vi "Acquire.vi"(8 "error in (no error)":errorcluster, 11 "ATS9350 in":refnum<class "ATS9350.lvclass">) -> (0 "error out":errorcluster, 3 "ATS9350 out":refnum<class "ATS9350.lvclass">)   [LabVIEW 2014, in "ATS9350.lvclass"]
uses:
  ATS9350.lvclass
  ATS-VI/ATS_ctl/ATS_Async_Ctrl.ctl
  DAQ Control Functional Global States.ctl
  DAQ Status States.ctl
  DAQ Class.lvclass
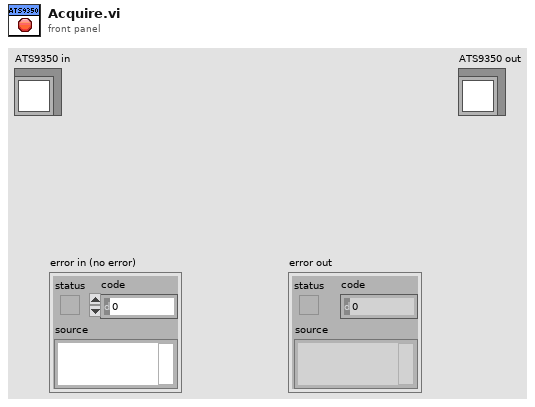
[diagram p1: front panel]
types:
  T1 = typedef "DAQ Control Functional Global States.ctl" = enum16{"Status", "Set Processing Finished", "Reset", "Clear", "Set DAQ Finished"}
  T2 = typedef "ATS_Async_Ctrl.ctl" = enum16{"SetupDMA", "StartCapture", "Get", "Get_Stream", "Abort", "Stop"}
  T3 = typedef "DAQ Status States.ctl" = enum16{"Get", "Show"}
  T4 = typedef "ATS_Async_Status.ctl" = cluster{"Start DMA":bool, "StartCapture":bool, "Valid":bool, "Completed":bool, "InProgress":bool, "Timeout":bool, "Overflow":bool, "Error":bool}
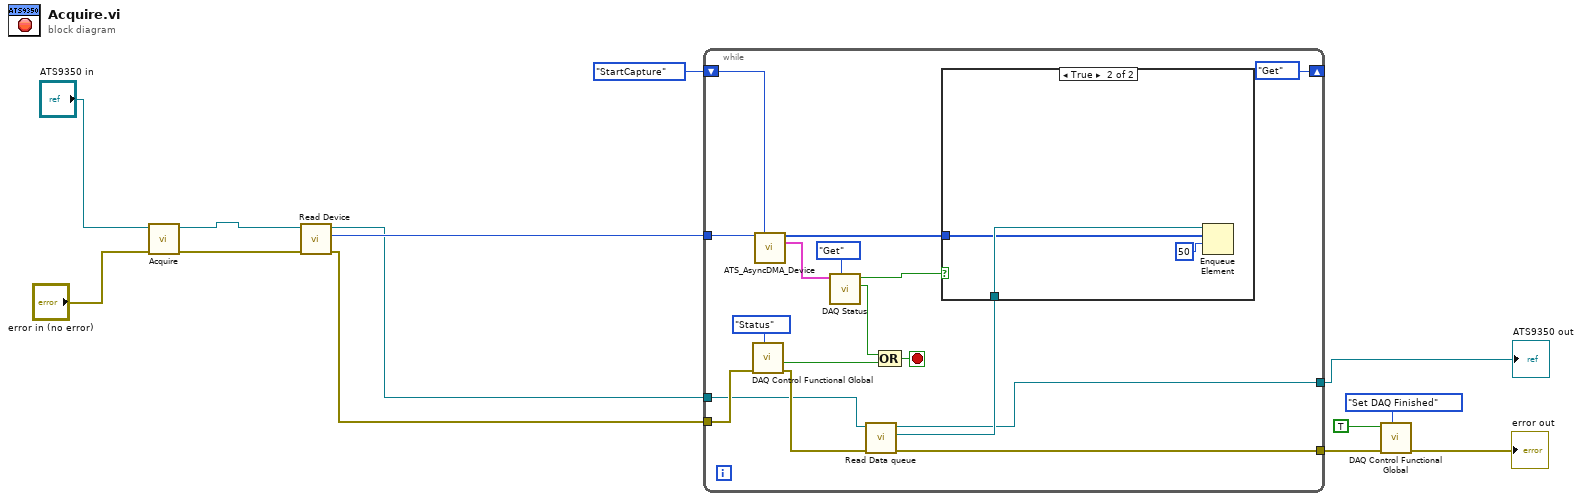
[diagram p0: block diagram]
diagram:
  n1 = call-parent "Acquire.vi"("error in (no error)"="error in (no error)", "DAQ Class in"="ATS9350 in") -> ("error out"=w1:errorcluster, "DAQ Class out"=w2:refnum<class "ATS9350.lvclass">)  [unwired: 8 in]
  n2 = call-dynamic "Read Device.vi"("error in (no error)"=w1, "ATS9350 in"=w2) -> ("error out"=w9:errorcluster, "Device"=w11:i32, "ATS9350 out"=w10:refnum<class "ATS9350.lvclass">)  [unwired: 7 in]
  n3 = while {
    tunnel: w11 -> [w30]
    shift-right: [ATS_Async_Ctrl."Get" ("ATS_Async_Ctrl")] -> _
    shift-left: ATS_Async_Ctrl."StartCapture" ("ATS_Async_Ctrl") -> [w29]
    tunnel: w10 -> [w16]
    tunnel: w9 -> [w19]
    tunnel: [w21] -> w3
    tunnel: [w15] -> w7
    stop <- w20 stop-if-true
    n4 = call "DAQ Control Functional Global.vi"("State"=DAQ_Control_Functional_Global_States."Status", "Error In"=w19) -> ("Error Out"=w17:errorcluster, "Reset?"=w18:bool)  [unwired: 6 in, 2 out]
    n5 = call "ATS_AsyncDMA_Device.vi"("DeviceIn"=w30, "ATS_Async_Ctrl"=w29) -> ("Buffer"=w27:u16[], "Async_Status"=w26:T4)  [unwired: 9 in, 3 out]
    n6 = call "DAQ Status.vi"("Enum"=DAQ_Status_States."Get", "Async_Status"=w26) -> ("DAQ Error?"=w22:bool, "Valid"=w25:bool)  [unwired: 8 in]
    n7 = call-dynamic "Read Data queue.vi"("error in (no error)"=w17, "DAQ Class in"=w16) -> ("error out"=w15:errorcluster, "Data queue"=w23:refnum<queue>, "DAQ Class out"=w21:refnum<class "ATS9350.lvclass">)  [unwired: 7 in]
    n8 = Compound Arithmetic op=OR(w22, w18) -> (w20:bool)
    n9 = case shown="True" w25 {
      tunnel: w27 -> [_ w31]
      tunnel: w23 -> [_ w33]
      frame False {
        # "Do nothing"
      }
      frame True {
        n10 = Enqueue Element(queue=w33, element=w31, timeout in ms (-1)=50) -> ()  [unwired: 1 in, 3 out]
      }
    }
  }
  "ATS9350 out" <- w3
  n11 = call "DAQ Control Functional Global.vi"("State"=DAQ_Control_Functional_Global_States."Set DAQ Finished", "Error In"=w7, "DAQ Finished In"=TRUE) -> ("Error Out"=→"error out":errorcluster)  [unwired: 5 in, 3 out]
